vi "niRFUtil INC GBL Validate Settings Flag.vi"() -> ()   [LabVIEW 2015, in "niRFUtil.lvlib"]
uses:
  niRFUtil.lvlib
  niRFUtil INC Validate Settings Enabled.ctl
panel:
  in  "Validation Enabled":T1=enum."True"
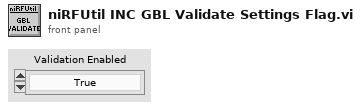
[diagram p1: front panel]
types:
  T1 = typedef "niRFUtil.lvlib/niRFUtil INC Validate Settings Enabled.ctl" = enum16{"False", "True"}
diagram:
